vi "PSPOP_Update Cell String.vi"(8 "error in (no error)":errorcluster, 9 "Call Data (must be Cell Info cluster)":variant, 11 "Popup Value":variant) -> (0 "error out":errorcluster, 1 "Cell Data":variant)   [LabVIEW 2016]
uses:
  Private/Ctrls/PSPOP_Grid.Cell Info.ctl
  Private/Ctrls/POP_Data Type.ctl
panel:
  in  "rect":T1
  in  "point":cluster{"x":i16, "y":i16}
  in  "Cell Info (type only)":T2={"Tag"="", "Row"=0, "Column"=0, "In Symbol?"=FALSE, "In Data?"=FALSE, "Cell String"="", "Ctl Refnum"=refnum, "Prop Type"=enum."Unkown", "Ring Strings"=[], "Ring Values"=[], "New Cell String"=""}
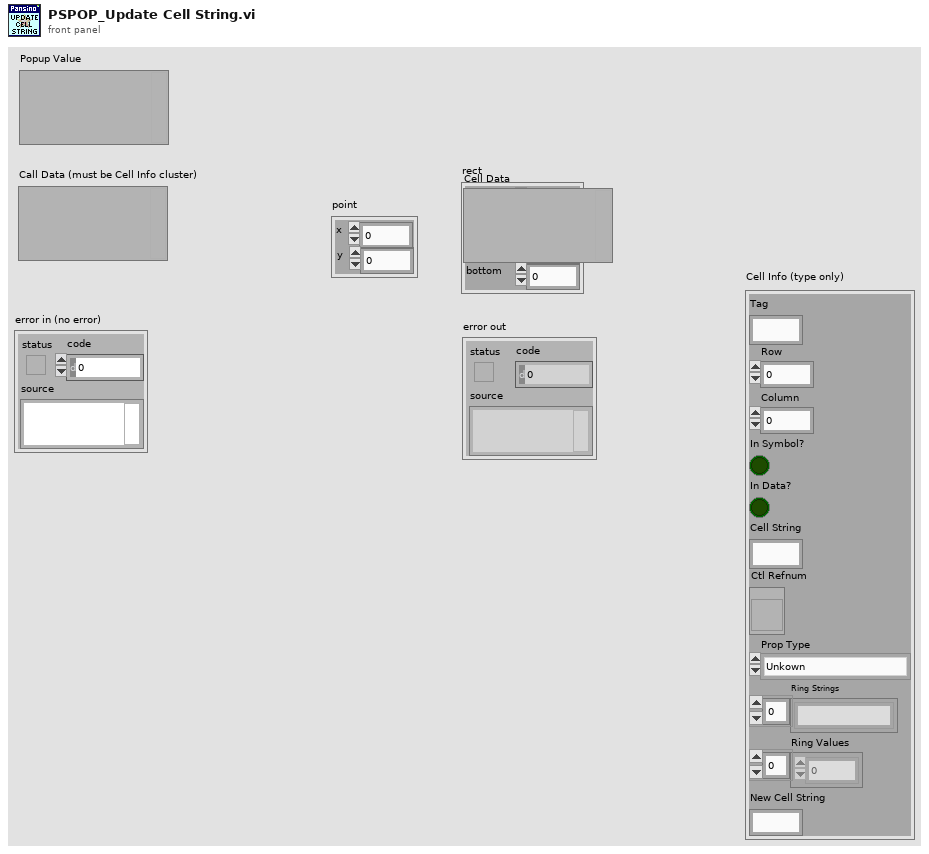
[diagram p1: front panel]
types:
  T1 = cluster{"left":i16, "top":i16, "right":i16, "bottom":i16}
  T2 = typedef "PSPOP_Grid.Cell Info.ctl" = cluster{"Tag":string, "Row":i32, "Column":i32, "In Symbol?":bool, "In Data?":bool, "Cell String":string, "Ctl Refnum":refnum<vi>, "Prop Type":T3, "Ring Strings":string[], "Ring Values":ext[], "New Cell String":string}
  T3 = typedef "POP_Data Type.ctl" = enum16{"NO POPUP", "Unkown", "String", "Integer", "Float", "Color", "Boolean", "Ring", "Captioned String", "Captioned Integer", "Button Color", "2 Int Cluster", "4 Int Cluster", "6-Dbl Cluster", "Path", "Combox", "Time", "ShotCut String"}
  T4 = cluster{"a0":i32, "a1":i32, "a2":i32, "a3":i32, "a4":i32, "a5":i32}
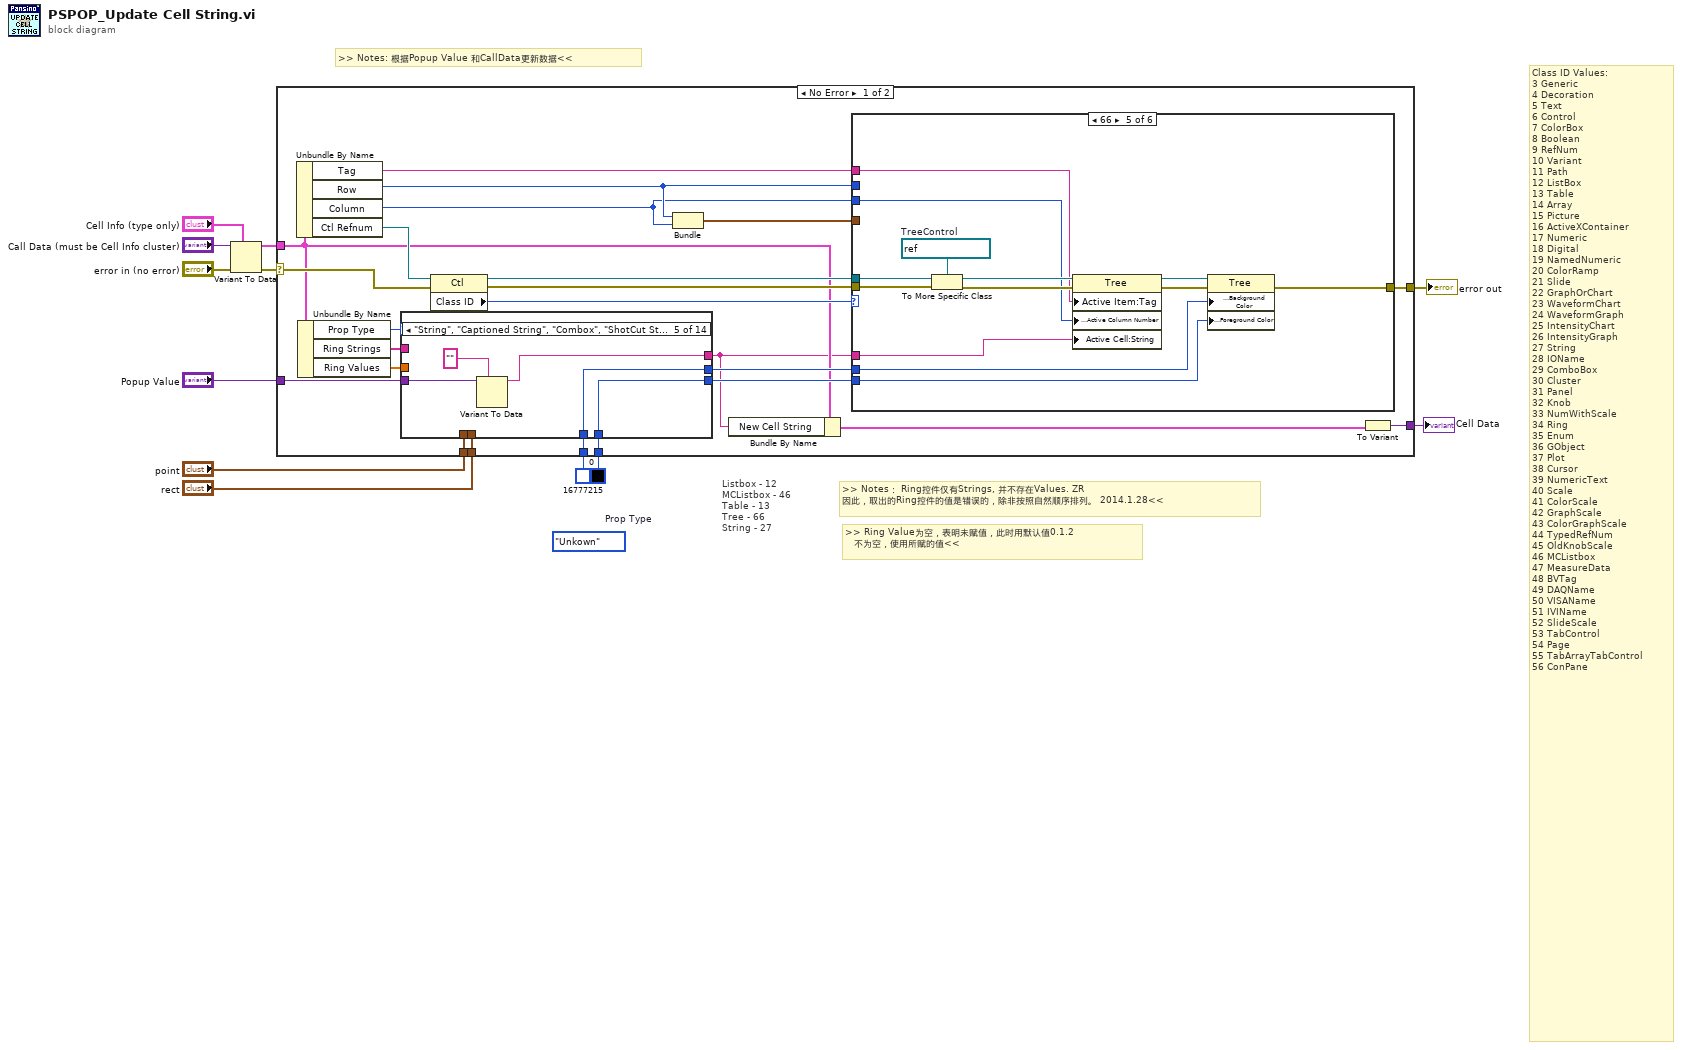
[diagram p0: block diagram]
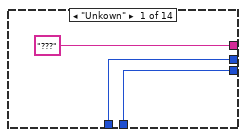
[diagram p2: hidden frame]
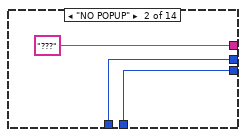
[diagram p3: hidden frame]
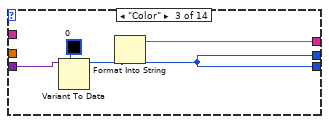
[diagram p4: hidden frame]
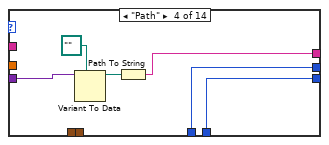
[diagram p5: hidden frame]
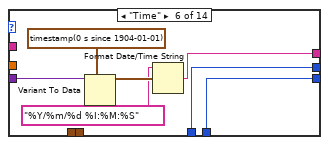
[diagram p6: hidden frame]
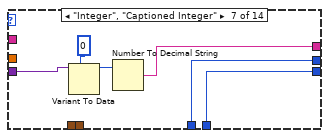
[diagram p7: hidden frame]
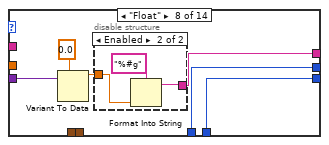
[diagram p8: hidden frame]
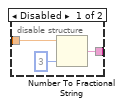
[diagram p9: hidden frame]
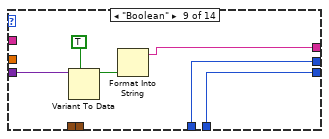
[diagram p10: hidden frame]
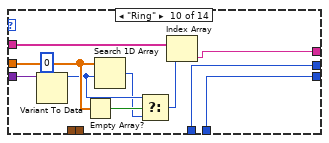
[diagram p11: hidden frame]
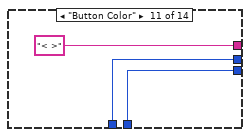
[diagram p12: hidden frame]
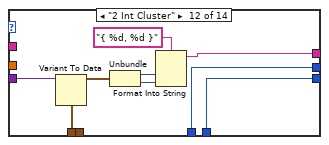
[diagram p13: hidden frame]
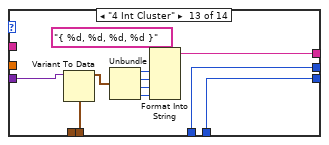
[diagram p14: hidden frame]
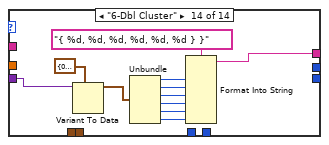
[diagram p15: hidden frame]
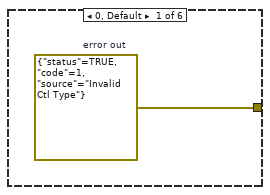
[diagram p16: hidden frame]
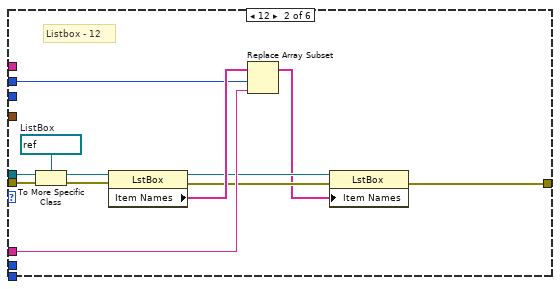
[diagram p17: hidden frame]
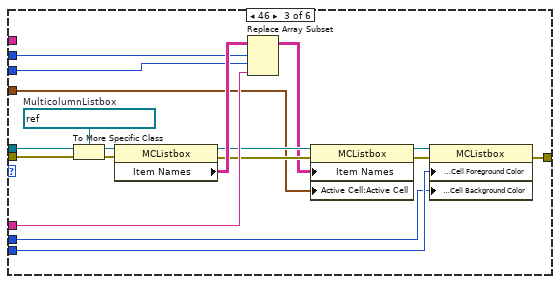
[diagram p18: hidden frame]
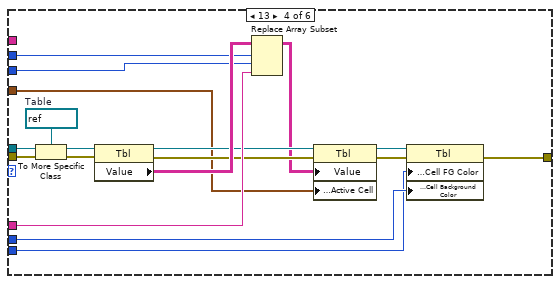
[diagram p19: hidden frame]
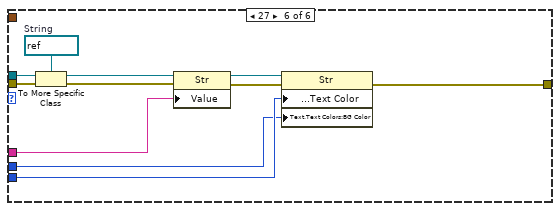
[diagram p20: hidden frame]
diagram:
  (unwired) POP_Data_Type."Unkown"  # Prop Type
  # ">> Ring Value为空，表明未赋值，此时用默认值0.1.2\n   不为空，使用所赋的值<<"
  # ">> Notes: 根据Popup Value 和CallData更新数据<<"
  # "Class ID Values:\n3 Generic \n4 Decoration \n5 Text \n6 Control \n7 ColorBox \n8 Boolean \n9 RefNum \n10 Variant \n11 Path \n12 ListBox \n13 Table \n14 Array \n15 Picture \n16 ActiveXContainer \n17 Numeric \n18 Digital \n19 NamedNumeric \n20 ColorRamp \n21 Slide \n22 GraphOrChart \n23 WaveformChart \n24 WaveformGraph \n25 IntensityChart \n26 IntensityGraph \n27 String \n28 IOName \n29 ComboBox \n30 Cluster \n31 Panel \n32 Knob \n33 NumWithScale \n34 Ring \n35 Enum \n36 GObject \n37 Plot \n38 Cursor \n39 NumericText \n40 Scale \n41 ColorScale \n42 GraphScale \n43 ColorGraphScale \n44 TypedRefNum \n45 OldKnobScale \n46 MCListbox \n47 MeasureData \n48 BVTag \n49 DAQName \n50 VISAName \n51 IVIName \n52 SlideScale \n53 TabControl \n54 Page \n55 TabArrayTabControl \n56 ConPane"
  # "Listbox - 12\nMCListbox - 46\nTable - 13\nTree - 66\nString - 27"
  # ">> Notes： Ring控件仅有Strings, 并不存在Values. ZR\n因此，取出的Ring控件的值是错误的，除非按照自然顺序排列。 2014.1.28<<"
  n1 = Variant To Data(error in="error in (no error)", type="Cell Info (type only)", Variant="Call Data (must be Cell Info cluster)") -> (data=w10:T2, error out=w8:errorcluster)
  n2 = case shown="No Error" w8 {
    selector: w8 -> [w18 _]
    tunnel: w10 -> [w17 _]
    tunnel: [w32 w207] -> w9
    tunnel: "Popup Value" -> [w30 _]
    tunnel: "point" -> [w29 _]
    tunnel: "rect" -> [w28 _]
    tunnel: u32 0 -> [w24 _]
    tunnel: u32 16777215 -> [w23 _]
    tunnel: [w14 _] -> w1
    frame No Error {
      n3 = Unbundle By Name(w17) -> ("Tag"=w33:string, "Row"=w22:i32, "Column"=w21:i32, "Ctl Refnum"=w19:refnum<vi>)
      n4 = Unbundle By Name(w17) -> ("Prop Type"=w27:T3, "Ring Strings"=w31:string[], "Ring Values"=w13:ext[])
      n5 = case shown="\"String\", \"Captioned String\", \"Combox\", \"ShotCut String\"" w27 {
        tunnel: w31 -> [_ _ _ _ _ _ _ _ _ w97 _ _ _ _]
        tunnel: w30 -> [_ _ w46 w52 w54 w62 w68 w74 w86 w99 _ w111 w122 w124]
        tunnel: ["???" "???" w44 w47 w53 w58 w65 w71 w83 w96 "< >" w105 w118 w123] -> w16
        tunnel: w29 -> [_ _ _ _ _ _ _ _ _ _ _ w110 _ _]
        tunnel: w28 -> [_ _ _ _ _ _ _ _ _ _ _ _ w117 _]
        tunnel: [w37 w40 w43 w50 w57 w64 w70 w76 w88 w94 w100 w104 w113 _] -> w26
        tunnel: [w38 w41 w43 w51 w56 w63 w69 w75 w87 w95 w101 w103 w112 _] -> w25
        tunnel: w24 -> [w37 w40 _ w50 w57 w64 w70 w76 w88 w94 w100 w104 w113 _]
        tunnel: w23 -> [w38 w41 _ w51 w56 w63 w69 w75 w87 w95 w101 w103 w112 _]
        tunnel: w13 -> [_ _ _ _ _ _ _ _ _ w93 _ _ _ _]
        frame "Unkown" {
        }
        frame "NO POPUP" {
        }
        frame "Color" {
          n6 = Variant To Data(type=u32 0, Variant=w46) -> (data=w43:u32)  [unwired: 1 in, 1 out]
          n7 = Format Into String(w43) -> (resulting string=w44:string)  [unwired: 3 in, 1 out]
        }
        frame "Path" {
          n8 = Variant To Data(type=path "", Variant=w52) -> (data=w48:path)  [unwired: 1 in, 1 out]
          n9 = Path To String(path=w48) -> (string=w47:string)
        }
        frame "String", "Captioned String", "Combox", "ShotCut String" {
          n10 = Variant To Data(type="", Variant=w54) -> (data=w53:string)  [unwired: 1 in, 1 out]
        }
        frame "Time" {
          n11 = Variant To Data(type=timestamp(0 s since 1904-01-01) ("Time"), Variant=w62) -> (data=w60:timestamp)  [unwired: 1 in, 1 out]
          n12 = Format Date/Time String(time format string (%c)="%Y/%m/%d %I:%M:%S" ("时间格式字符串(%c)"), seconds (now)=w60) -> (date/time string=w58:string)  [unwired: 1 in]
        }
        frame "Integer", "Captioned Integer" {
          n13 = Variant To Data(type=0, Variant=w68) -> (data=w66:i32)  [unwired: 1 in, 1 out]
          n14 = Number To Decimal String(number=w66) -> (decimal integer string=w65:string)  [unwired: 1 in]
        }
        frame "Float" {
          n15 = Variant To Data(type=0.0, Variant=w74) -> (data=w72:dbl)  [unwired: 1 in, 1 out]
          n16 = disable-structure shown="Enabled" {
            disable-tunnel: w72 -> [w79 w81]
            disable-tunnel: [w78 w80] -> w71
            frame Disabled {
              n17 = Number To Fractional String(number=w79, precision (6)=i16 3 ("精度(6)")) -> (F-format string=w78:string)  [unwired: 2 in]
            }
            frame Enabled {
              n18 = Format Into String(format string="%#g" ("initial string"), w81) -> (resulting string=w80:string)  [unwired: 2 in, 1 out]
            }
          }
        }
        frame "Boolean" {
          n19 = Variant To Data(type=TRUE, Variant=w86) -> (data=w84:bool)  [unwired: 1 in, 1 out]
          n20 = Format Into String(w84) -> (resulting string=w83:string)  [unwired: 3 in, 1 out]
        }
        frame "Ring" {
          n21 = Variant To Data(type=0, Variant=w99) -> (data=w91:i32)  [unwired: 1 in, 1 out]
          n22 = Empty Array?(array=w93) -> (empty?=w92:bool)
          n23 = Search 1D Array(1D array=w93, element=w91) -> (index of element=w90:i32)  [unwired: 1 in]
          n24 = Select(t=w91, s=w92, f=w90) -> (s? t:f=w89:i32)
          n25 = Index Array(array=w97, index=w89) -> (element=w96:string)
        }
        frame "Button Color" {
        }
        frame "2 Int Cluster" {
          n26 = Variant To Data(type=w110, Variant=w111) -> (data=w106:cluster{"x":i16, "y":i16})  [unwired: 1 in, 1 out]
          n27 = Unbundle(w106) -> ("x"=w108:i16, "y"=w107:i16)
          n28 = Format Into String(format string="{ %d, %d }" ("String"), w108, w107) -> (resulting string=w105:string)  [unwired: 2 in, 1 out]
        }
        frame "4 Int Cluster" {
          n29 = Variant To Data(type=w117, Variant=w122) -> (data=w119:T1)  [unwired: 1 in, 1 out]
          n30 = Unbundle(w119) -> ("left"=w121:i16, "top"=w120:i16, "right"=w116:i16, "bottom"=w115:i16)
          n31 = Format Into String(format string="{ %d, %d, %d, %d }" ("String"), w121, w120, w116, w115) -> (resulting string=w118:string)  [unwired: 2 in, 1 out]
        }
        frame "6-Dbl Cluster" {
          n32 = Variant To Data(type=T4 {"a0"=0, "a1"=0, "a2"=0, "a3"=0, "a4"=0, "a5"=0} ("rect"), Variant=w124) -> (data=w131:T4)  [unwired: 1 in, 1 out]
          n33 = Unbundle(w131) -> ("a0"=w133:i32, "a1"=w132:i32, "a2"=w130:i32, "a3"=w129:i32, "a4"=w126:i32, "a5"=w125:i32)
          n34 = Format Into String(format string="{ %d, %d, %d, %d, %d, %d } }" ("String"), w133, w132, w130, w129, w126, w125) -> (resulting string=w123:string)  [unwired: 2 in, 1 out]
        }
      }
      n35 = property class="Ctl"(reference=w19, error in=w18) -> (reference out=w35:refnum<vi>, error out=w34:errorcluster, "Class ID"=w36:u32)
      n36 = Bundle("Row"=w22, "Column"=w21) -> (w20:cluster{"Row":i32, "Column":i32})  [unwired: 1 in]
      n37 = Bundle By Name(cluster=w17, "New Cell String"=w16) -> (w15:T2)
      n38 = case shown="66" w36 {
        tunnel: w35 -> [_ w145 w163 w181 w194 w205]
        tunnel: w34 -> [_ w144 w162 w180 w193 w204]
        tunnel: w16 -> [_ w140 w158 w176 w188 w201]
        tunnel: w22 -> [_ w136 w154 w172 _ _]
        tunnel: w21 -> [_ _ w153 w171 w189 _]
        tunnel: w33 -> [_ _ _ _ w190 _]
        tunnel: [w134 w135 w147 w165 w183 w196] -> w32
        tunnel: w26 -> [_ _ w150 w167 w186 w199]
        tunnel: w25 -> [_ _ w149 w168 w185 w198]
        tunnel: w20 -> [_ _ w152 w170 _ _]
        frame 0, Default {
          w134 = errorcluster {"status"=TRUE, "code"=1, "source"="Invalid Ctl Type"}  # error out
        }
        frame 12 {
          w146 = refnum<vi> refnum  # ListBox
          # "Listbox - 12"
          n39 = To More Specific Class(target class=w146, reference=w145, error in=w144) -> (specific class reference=w143:refnum<vi>, error out=w142:errorcluster)
          n40 = property class="LstBox"(reference=w143, error in=w142) -> (reference out=w139:refnum<vi>, error out=w138:errorcluster, "Item Names"=w141:string[])
          n41 = Replace Array Subset(array=w141, new element=w140, index=w136) -> (w137:string[])
          n42 = property class="LstBox"(reference=w139, error in=w138, "Item Names"=w137) -> (error out=w135:errorcluster)  [unwired: 1 out]
        }
        frame 46 {
          w164 = refnum<vi> refnum  # MulticolumnListbox
          n43 = To More Specific Class(target class=w164, reference=w163, error in=w162) -> (specific class reference=w161:refnum<vi>, error out=w160:errorcluster)
          n44 = property class="MCListbox"(reference=w161, error in=w160) -> (reference out=w157:refnum<vi>, error out=w156:errorcluster, "Item Names"=w159:string[][])
          n45 = Replace Array Subset(array=w159, new element=w158, index (row)=w154, index (col)=w153) -> (w155:string[][])
          n46 = property class="MCListbox"(reference=w157, error in=w156, "Item Names"=w155, "Active Cell:Active Cell"=w152) -> (reference out=w151:refnum<vi>, error out=w148:errorcluster)
          n47 = property class="MCListbox"(reference=w151, error in=w148, "Active Cell:Cell Foreground Color"=w150, "Active Cell:Cell Background Color"=w149) -> (error out=w147:errorcluster)  [unwired: 1 out]
        }
        frame 13 {
          w182 = refnum<vi> refnum  # Table
          n48 = To More Specific Class(target class=w182, reference=w181, error in=w180) -> (specific class reference=w179:refnum<vi>, error out=w178:errorcluster)
          n49 = property class="Tbl"(reference=w179, error in=w178) -> (reference out=w175:refnum<vi>, error out=w174:errorcluster, "Value"=w177:string[][])
          n50 = Replace Array Subset(array=w177, new element=w176, index (row)=w172, index (col)=w171) -> (w173:string[][])
          n51 = property class="Tbl"(reference=w175, error in=w174, "Value"=w173, "Active Cell:Active Cell"=w170) -> (reference out=w169:refnum<vi>, error out=w166:errorcluster)
          n52 = property class="Tbl"(reference=w169, error in=w166, "Active Cell:Cell FG Color"=w167, "Active Cell:Cell Background Color"=w168) -> (error out=w165:errorcluster)  [unwired: 1 out]
        }
        frame 66 {
          w195 = refnum<vi> refnum  # TreeControl
          n53 = To More Specific Class(target class=w195, reference=w194, error in=w193) -> (specific class reference=w192:refnum<vi>, error out=w191:errorcluster)
          n54 = property class="Tree"(reference=w192, error in=w191, "Active Item:Tag"=w190, "Active Cell:Active Column Number"=w189, "Active Cell:String"=w188) -> (reference out=w187:refnum<vi>, error out=w184:errorcluster)
          n55 = property class="Tree"(reference=w187, error in=w184, "Active Cell:Background Color"=w185, "Active Cell:Foreground Color"=w186) -> (error out=w183:errorcluster)  [unwired: 1 out]
        }
        frame 27 {
          w206 = refnum<vi> refnum  # String
          n56 = To More Specific Class(target class=w206, reference=w205, error in=w204) -> (specific class reference=w203:refnum<vi>, error out=w202:errorcluster)
          n57 = property class="Str"(reference=w203, error in=w202, "Value"=w201) -> (reference out=w200:refnum<vi>, error out=w197:errorcluster)
          n58 = property class="Str"(reference=w200, error in=w197, "Text.Text Colors:Text Color"=w199, "Text.Text Colors:BG Color"=w198) -> (error out=w196:errorcluster)  [unwired: 1 out]
        }
      }
      n59 = To Variant(anything=w15) -> (Variant=w14:variant)
    }
    frame Error {
      w207 = errorcluster {"status"=TRUE, "code"=1, "source"="Invalid Call Data"}  # error out
    }
  }
  "error out" <- w9
  "Cell Data" <- w1
